vi "GetPanVIRef.vi"(8 "error in (no error)":errorcluster caption="entrée d'erreur (pas d'erreur)", 11 "BaseDevice en entrée":refnum<class "BaseDevice.lvclass"> caption="DNL_LabVIEW Object in") -> (0 "error out":errorcluster caption="sortie d'erreur", 1 "ClassName":string, 2 "PanelVIRef":refnum<vi>, 3 "BaseDevice en sortie":refnum<class "BaseDevice.lvclass"> caption="DNL_LabVIEW Object out")   [LabVIEW 2019, in "BaseDevice.lvclass"]
uses:
  BaseDevice.lvclass
  BaseDevice.lvclass/BaseDevice.ctl
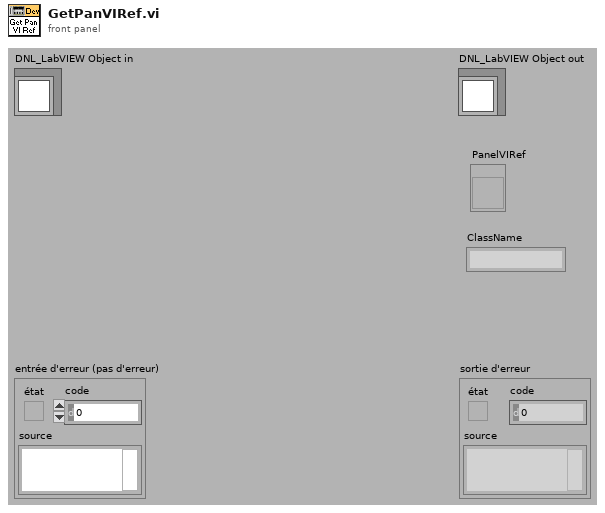
[diagram p1: front panel]
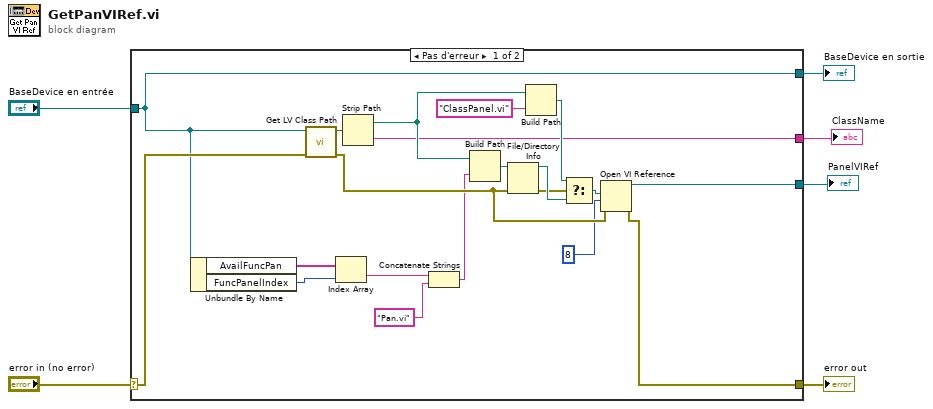
[diagram p0: block diagram]
diagram:
  n1 = case shown="Pas d'erreur" "error in (no error)" {
    selector: "error in (no error)" -> [w15 w28]
    tunnel: [w13 w28] -> w5
    tunnel: [w11 w27] -> w3
    tunnel: "BaseDevice en entrée" -> [w11 w27]
    tunnel: [w14 _] -> w2
    tunnel: [w12 _] -> w1
    frame No Error {
      n2 = Unbundle By Name(w11) -> ("AvailFuncPan"=w10:string[], "FuncPanelIndex"=w9:i32)
      n3 = call <vilib>:"Get LV Class Path.vi"("error in (no error)"=w15, "object"=w11) -> ("error out"=w25:errorcluster, "class path"=w16:path)  [unwired: 8 in]
      n4 = Index Array(array=w10, index=w9) -> (element=w8:string)
      n5 = Strip Path(path=w16) -> (stripped path=w21:path, name=w14:string)
      n6 = Concatenate Strings(w8, "Pan.vi" ("nom ou chemin relatif")) -> (w18:string)
      n7 = Build Path(base path=w21, name or relative path=w18) -> (appended path=w19:path)
      n8 = File/Directory Info(path=w19, error in=w25) -> (path out=w24:path, error out=w20:errorcluster)  [unwired: 5 out]
      n9 = Build Path(base path=w21, name or relative path="ClassPanel.vi") -> (appended path=w23:path)
      n10 = Select(t=w23, s=w20, f=w24) -> (s? t:f=w26:path)
      n11 = Open VI Reference(vi path=w26, options=8, error in (no error)=w25) -> (vi reference=w12:refnum<vi>, error out=w13:errorcluster)  [unwired: 3 in]
    }
    frame Error {
    }
  }
  "error out" <- w5
  "BaseDevice en sortie" <- w3
  "ClassName" <- w2
  "PanelVIRef" <- w1
